vi "DEBUG_LEVEL - Type.vi"(8 "error in (no error)":errorcluster) -> (0 "error out":errorcluster, 3 "DEBUG_LEVEL_VALUE":i32)   [LabVIEW 2013]
doc: "<b>Buffer policy settings can be only unsafe in xiAPI LabVIEW library</b>\nUNSAFE : User gets pointer to internally allocated circle buffer and data may be overwritten by device.\nSAFE : Data from device will be copied to user allocated buffer or xiApi allocated memory."
uses:
  DEBUG_LEVEL.ctl
  C:/Projects/Cameras3.x/xiLib/xiLIB_64bit/xiLIB/xiCamLib/API/x64/xiApi.NETX64.dll
  xiLIB_64bit/xiLIB/xiCamLib/API/x64/xiApi.NETX64.dll
panel:
  in  "DEBUG_LEVEL":T1
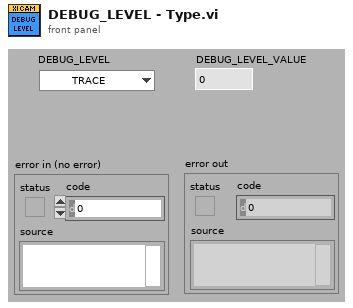
[diagram p1: front panel]
types:
  T1 = typedef "DEBUG_LEVEL.ctl" = enum16{"TRACE", "WARNING", "ERROR", "FATAL"}
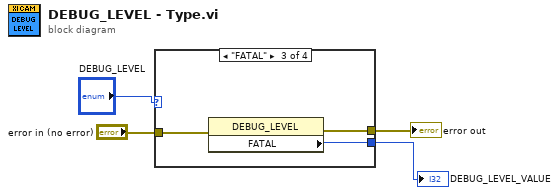
[diagram p0: block diagram]
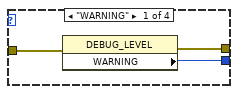
[diagram p2: hidden frame]
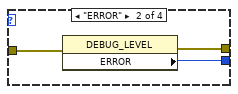
[diagram p3: hidden frame]
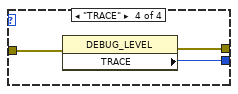
[diagram p4: hidden frame]
diagram:
  n1 = case shown="\"FATAL\"" "DEBUG_LEVEL" {
    tunnel: "error in (no error)" -> [w7 w10 w13 w16]
    tunnel: [w6 w9 w12 w15] -> w3
    tunnel: [w5 w8 w11 w14] -> w2
    frame "WARNING" {
      n2 = property class="DEBUG_LEVEL"(error in=w7) -> (error out=w6:errorcluster, "WARNING"=w5:i32)  [unwired: 1 in, 1 out]
    }
    frame "ERROR" {
      n3 = property class="DEBUG_LEVEL"(error in=w10) -> (error out=w9:errorcluster, "ERROR"=w8:i32)  [unwired: 1 in, 1 out]
    }
    frame "FATAL" {
      n4 = property class="DEBUG_LEVEL"(error in=w13) -> (error out=w12:errorcluster, "FATAL"=w11:i32)  [unwired: 1 in, 1 out]
    }
    frame "TRACE" {
      n5 = property class="DEBUG_LEVEL"(error in=w16) -> (error out=w15:errorcluster, "TRACE"=w14:i32)  [unwired: 1 in, 1 out]
    }
  }
  "error out" <- w3
  "DEBUG_LEVEL_VALUE" <- w2
